vi "Tracker.vi"(6 "error in":errorcluster, 7 "XYZdata in":dbl[][][](array[numeric])) -> (1 "frame":i32, 4 "error in 2":errorcluster, 5 "XYZdata out":dbl[][][](array[numeric]))   [LabVIEW 2011]
panel:
  in  "Xcor1D iterations":i32=1
  in  "QI iterations":i32=4
  out "Waveform Graph":sgl[](graph)
  in  "Enable tracking?":bool=TRUE
  out "Intensity Graph":sgl[][](graph)
  out "beads/s":dbl
  out "JTracker radial profile":sgl[](graph)
  out "QI pos":cluster{"X":sgl, "Y":sgl}(graph)
  out "Bead":i32
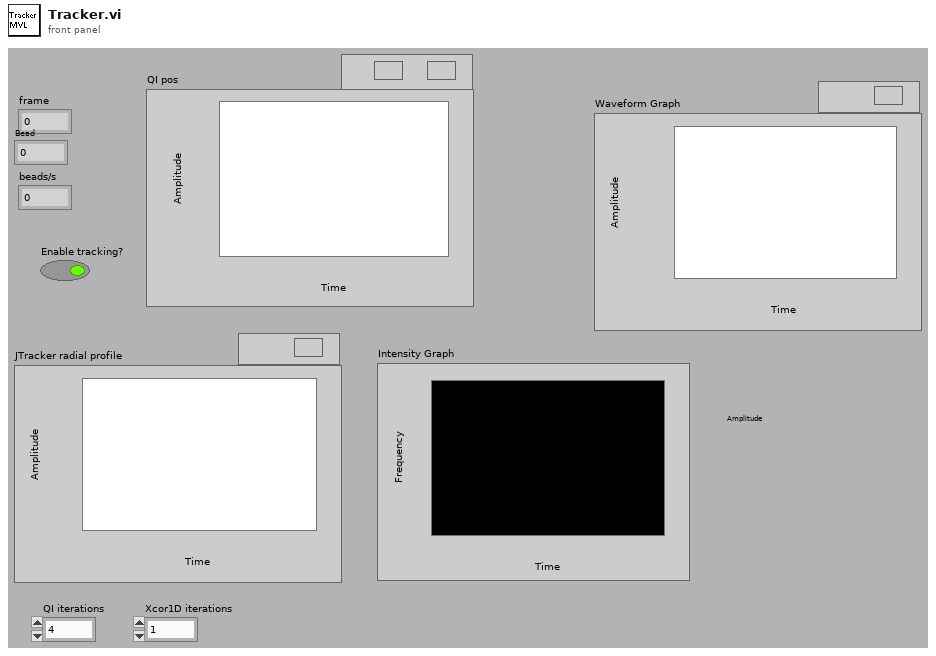
[diagram p1: front panel]
types:
  T1 = cluster{"Image Pixels (U8)":u8[][], "xy out":dbl[], "relative frame #":i32, "bead #":i32, "state":i32, "frame number":i32, "frame time":i32}
  T2 = cluster{"ROI1":i32, "Rmax (pix)":i32, "RminZ (pix)":i32, "LUTs":dbl[][][], "use trace":bool, "angular pixel\n coverage factor":dbl, "radial pixel\n coverage factor":dbl}
  T3 = typedef "TrackerInstance.ctl" = cluster{"Tracker Pointer":u64, "Image size":cluster{"width":u32, "height":u32}}
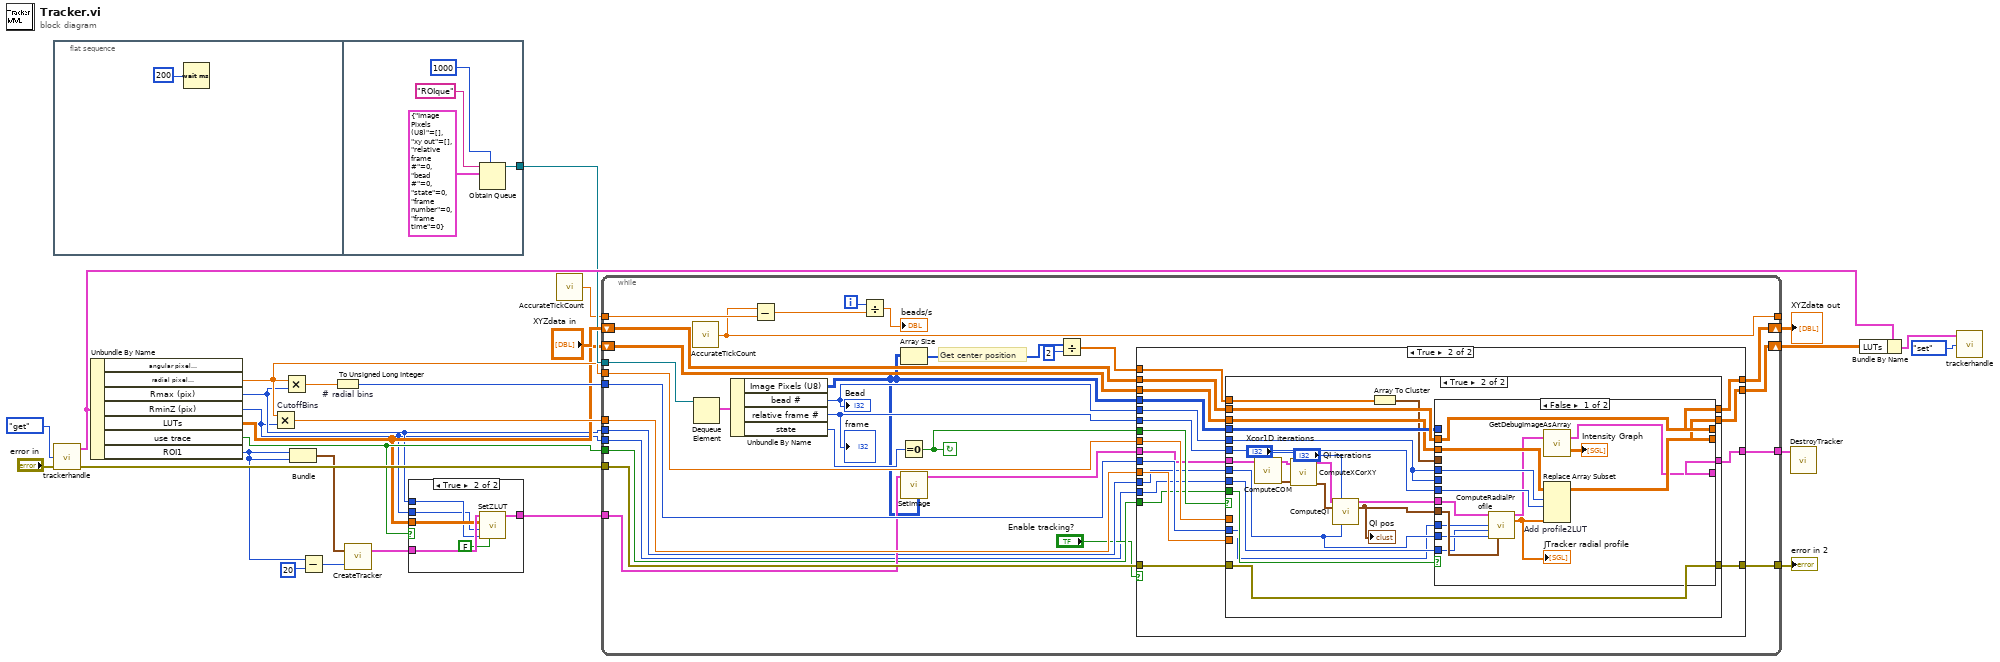
[diagram p0: block diagram]
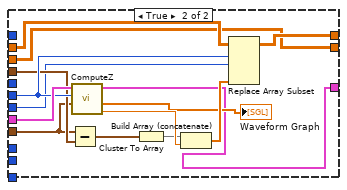
[diagram p5: hidden frame]
diagram:
  n1 = flat-sequence {
    tunnel: [w30] -> w17
    frame #0 {
      n2 = Wait (ms)(milliseconds to wait=u32 200) -> ()  [unwired: 1 out]
    }
    frame #1 {
      n3 = Obtain Queue(max queue size (-1, unlimited)=1000, name (unnamed)="ROIque", element data type=T1 {"Image Pixels (U8)"=[], "xy out"=[], "relative frame #"=0, "bead #"=0, "state"=0, "frame number"=0, "frame time"=0} ("output cluster")) -> (queue out=w30:refnum<queue>)  [unwired: 2 in, 2 out]
    }
  }
  n4 = call "trackerhandle.vi"("error in"="error in", "action"=enum16{"get", "set"}."get") -> ("error out"=w19:errorcluster, "output Cluster"=w23:T2)  [unwired: 1 in, 1 out]
  n5 = Unbundle By Name(w23) -> ("radial pixel\n coverage factor"=w14:dbl, "Rmax (pix)"=w3:i32, "RminZ (pix)"=w1:i32, "LUTs"=w4:dbl[][][], "use trace"=w7:bool, "ROI1"=w8:i32)  [unwired: 1 out]
  n6 = Multiply "CutoffBins"(x=w14, y=w1) -> (x*y=w13:dbl)
  n7 = Multiply(x=w14, y=w3) -> (x*y=w16:dbl)
  n8 = Bundle("ROI1"=w8, "ROI1"=w8) -> (w12:cluster{"ROI1":i32, "ROI1":i32})  [unwired: 1 in]
  n9 = Subtract(x=w8, y=20) -> (x-y=w9:i32)
  n10 = To Unsigned Long Integer "# radial bins"(number=w16) -> (unsigned 32bit integer=w15:u32)
  n11 = call "CreateTracker.vi"("XCorWindow"=w9, "Image size"=w12) -> ("tracker"=w6:T3)  [unwired: 1 in]
  n12 = case shown="True" w7 {
    tunnel: w6 -> [w33 w39]
    tunnel: [w33 w38] -> w5
    tunnel: w4 -> [_ w37]
    tunnel: w3 -> [_ w36]
    tunnel: w1 -> [_ w35]
    frame False {
    }
    frame True {
      n13 = call "SetZLUT.vi"("Compare with inner product"=FALSE ("Use correlation instead of least squared difference"), "maxradius"=w36, "minradius"=w35, "zluts"=w37, "tracker instance"=w39) -> ("tracker"=w38:T3)  [unwired: 5 in]
    }
  }
  n14 = call "AccurateTickCount.vi"() -> ("seconds"=w2:dbl)
  n15 = while {
    shift-right: [w69] -> w25
    shift-left: "XYZdata in" -> [w68]
    shift-right: [w67] -> w21
    shift-left: w4 -> [w66]
    tunnel: w19 -> [w60]
    tunnel: [w59] -> w18
    tunnel: w17 -> [w62]
    tunnel: w14 -> [w61]
    tunnel: w15 -> [w57]
    tunnel: w13 -> [w56]
    tunnel: w5 -> [w55]
    tunnel: [w53] -> w11
    tunnel: w7 -> [w52]
    tunnel: w3 -> [w51]
    tunnel: w2 -> [w44]
    tunnel: [w43] -> _
    tunnel: w1 -> [w40]
    i -> [w42]
    stop <- w63 continue-if-true
    # "Get center position"
    n16 = call "AccurateTickCount.vi"() -> ("seconds"=w43:dbl)
    n17 = Dequeue Element(queue=w62) -> (element=w70:T1)  [unwired: 1 in, 4 out]
    n18 = Unbundle By Name(w70) -> ("Image Pixels (U8)"=w47:u8[][], "bead #"=w64:i32, "relative frame #"=w58:i32, "state"=w65:i32)
    "frame" <- w58
    "Bead" <- w64
    n19 = Subtract(x=w43, y=w44) -> (x-y=w45:dbl)
    n20 = Divide(x=w42, y=w45) -> (x/y=→"beads/s":dbl)
    n21 = Array Size(array=w47) -> (size(s)=w49:i32[])
    n22 = Equal To 0?(x=w65) -> (x = 0?=w63:bool)
    n23 = call "SetImage.vi"("tracker"=w55, "Image (U8)"=w47) -> ("tracker"=w54:T3)  [unwired: 6 in, 1 out]
    n24 = Divide(x=w49, y=2) -> (x/y=w48:dbl[])
    n25 = case shown="True" "Enable tracking?" {
      tunnel: [w73 w93] -> w69
      tunnel: w68 -> [w73 w92]
      tunnel: [w72 w91] -> w67
      tunnel: w66 -> [w72 w90]
      tunnel: w64 -> [_ w89]
      tunnel: w63 -> [_ w88]
      tunnel: w61 -> [_ w87]
      tunnel: w60 -> [w74 w86]
      tunnel: [w74 w85] -> w59
      tunnel: w58 -> [_ w84]
      tunnel: w57 -> [_ w83]
      tunnel: w56 -> [_ w82]
      tunnel: w54 -> [w71 w81]
      tunnel: [w71 w80] -> w53
      tunnel: w52 -> [_ w79]
      tunnel: w51 -> [_ w78]
      tunnel: w48 -> [_ w77]
      tunnel: w47 -> [_ w76]
      tunnel: w40 -> [_ w75]
      frame False {
      }
      frame True {
        n26 = case shown="True" w88 {
          tunnel: [w97 w121] -> w93
          tunnel: w92 -> [w97 w120]
          tunnel: w89 -> [_ w119]
          tunnel: w84 -> [_ w118]
          tunnel: [w96 w117] -> w91
          tunnel: w90 -> [w96 w110]
          tunnel: w76 -> [_ w116]
          tunnel: w87 -> [_ _]
          tunnel: w86 -> [w95 w107]
          tunnel: [w95 w107] -> w85
          tunnel: w83 -> [_ w100]
          tunnel: w82 -> [_ _]
          tunnel: w81 -> [w94 w112]
          tunnel: [w94 w111] -> w80
          tunnel: w79 -> [_ w115]
          tunnel: w78 -> [_ w102]
          tunnel: w77 -> [_ w106]
          tunnel: w75 -> [_ w101]
          frame False {
          }
          frame True {
            n27 = call "ComputeCOM.vi"("tracker"=w112) -> ("position"=w113:cluster{"X":sgl, "Y":sgl}, "tracker"=w114:T3)  [unwired: 5 in]
            n28 = call "ComputeXCorXY.vi"("tracker"=w114, "iterations"="Xcor1D iterations", "position"=w113) -> ("tracker"=w109:T3, "position"=w108:cluster{"X":sgl, "Y":sgl})  [unwired: 2 in, 2 out]
            n29 = call "ComputeQI.vi"("tracker"=w109, "iterations"="QI iterations", "initial position"=w108, "maxRadius"=w102) -> ("tracker"=w103:T3, "position"=w104:cluster{"X":sgl, "Y":sgl})  [unwired: 9 in, 1 out]
            "QI pos" <- w104
            n30 = Array To Cluster(array=w106) -> (cluster=w105:cluster{"[0]":dbl, "[1]":dbl})
            n31 = case shown="False" w115 {
              tunnel: w120 -> [w135 w149]
              tunnel: w119 -> [_ w142]
              tunnel: [w135 w147] -> w121
              tunnel: w110 -> [w134 w146]
              tunnel: w119 -> [w133 _]
              tunnel: w118 -> [w132 w138]
              tunnel: [w131 w146] -> w117
              tunnel: w116 -> [_ _]
              tunnel: w103 -> [w128 w143]
              tunnel: [w125 w136] -> w111
              tunnel: w105 -> [_ w141]
              tunnel: w104 -> [w130 w139]
              tunnel: w102 -> [w129 _]
              tunnel: w101 -> [w123 _]
              tunnel: w100 -> [w122 _]
              frame False {
                n32 = call "ComputeRadialProfile.vi"("tracker"=w128, "radialsteps"=w122, "minradius"=w123, "maxradius"=w129, "center"=w130) -> ("tracker"=w127:T3, "output"=w126:sgl[])  [unwired: 8 in, 1 out]
                "JTracker radial profile" <- w126
                n33 = call "GetDebugImageAsArray.vi"("tracker"=w127) -> ("image"=→"Intensity Graph":sgl[][], "tracker"=w125:T3)  [unwired: 1 in]
                n34 = Replace Array Subset "Add profile2LUT"(array=w134, new element=w126, index (dim 0)=w133, index (dim 1)=w132) -> (w131:dbl[][][])  [unwired: 1 in]
              }
              frame True {
                n35 = Subtract(x=w139, y=w141) -> (x-y=w140:cluster{dbl, dbl})
                n36 = call "ComputeZ.vi"("position"=w139, "zlutIndex"=w142, "tracker instance"=w143) -> ("Z"=w145:sgl, "errorcurve"=→"Waveform Graph":sgl[], "tracker instance"=w136:T3)  [unwired: 4 in, 1 out]
                n37 = Cluster To Array(cluster=w140) -> (array=w144:dbl[])
                n38 = Build Array (concatenate)(w144, w145) -> (w148:dbl[])
                n39 = Replace Array Subset(array=w149, new element=w148, index (dim 0)=w142, index (dim 1)=w138) -> (w147:dbl[][][])  [unwired: 1 in]
              }
            }
          }
        }
      }
    }
  }
  "XYZdata out" <- w25
  "error in 2" <- w18
  n40 = call "DestroyTracker.vi"("tracker instance"=w11) -> ()  [unwired: 5 in]
  n41 = Bundle By Name(cluster=w23, "LUTs"=w21) -> (w22:T2)
  n42 = call "trackerhandle.vi"("action"=enum16{"get", "set"}."set", "input Cluster"=w22) -> ()  [unwired: 1 in, 3 out]
